vi "Increment.vi"(10 "boolean":bool, 11 "number in":u16) -> (3 "number out":u16)   [LabVIEW 2016]
doc: "increments number in by one if boolean is TRUE"
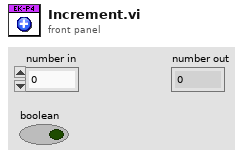
[diagram p1: front panel]
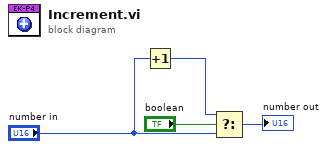
[diagram p0: block diagram]
diagram:
  n1 = Increment(x="number in") -> (x+1=w2:u16)
  n2 = Select(t=w2, s="boolean", f="number in") -> (s? t:f=→"number out":u16)
